vi "passIfError.vi"(6 "passing error codes (default = any error code)":i32[](array[numeric]), 7 "custom report message (\"\")":string, 8 "error in (no error)":errorcluster, 9 "task (\"\")":string, 10 "error":errorcluster, 11 "TestCase in":refnum<class "TestCase.lvclass">) -> (0 "error out":errorcluster, 3 "TestCase out":refnum<class "TestCase.lvclass">)   [LabVIEW 2011, in "TestCase.lvclass"]
doc: "Pass if 'error.status'=TRUE. 'error' is the error generated by the task. 'task' is the description of the task failure. 'error in' is for framework errors not related to the test task. 'passing error codes' can be used to define specific error codes that will cause the test to pass so that unexpected errors are still raised as test failures.\n\nUse this method when you want to test that an expected error is correctly raised."
uses:
  TestCase.lvclass
  TestCase.lvclass/TestCase.ctl
  JKI Reuse/Filter Error Codes (Array)__jki_lib_error_handling -- VI Tester.vi
panel:
  # "JKI VI Tester for LabVIEW\nhttp://jkisoft.com/vi-tester\nCopyright (C) 2007-2009, JKI <info@jkisoft.com>\nALL RIGHTS RESERVED"
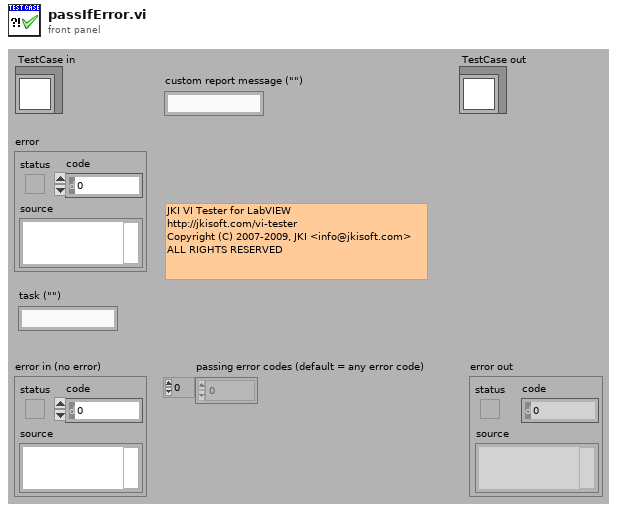
[diagram p1: front panel]
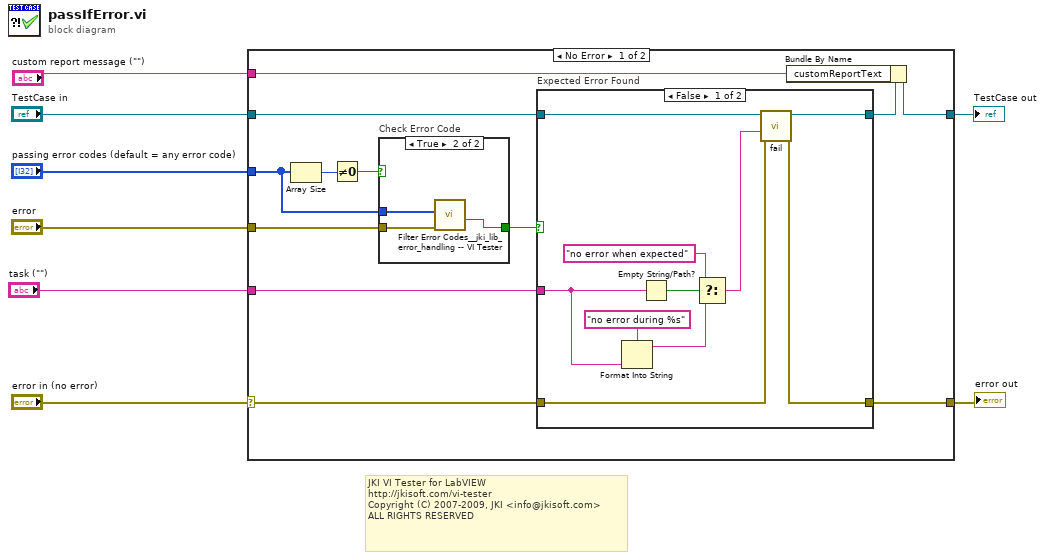
[diagram p0: block diagram]
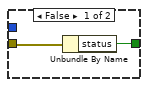
[diagram p2: hidden frame]
diagram:
  # "JKI VI Tester for LabVIEW\nhttp://jkisoft.com/vi-tester\nCopyright (C) 2007-2009, JKI <info@jkisoft.com>\nALL RIGHTS RESERVED"
  n1 = case shown="No Error" "error in (no error)" {
    selector: "error in (no error)" -> [w20 w39]
    tunnel: [w19 w39] -> w7
    tunnel: [w15 w38] -> w5
    tunnel: "TestCase in" -> [w18 w38]
    tunnel: "error" -> [w13 _]
    tunnel: "task (\"\")" -> [w17 _]
    tunnel: "custom report message (\"\")" -> [w14 _]
    tunnel: "passing error codes (default = any error code)" -> [w10 _]
    frame No Error {
      n2 = Array Size(array=w10) -> (size(s)=w9:i32)
      n3 = Not Equal To 0?(x=w9) -> (x != 0?=w12:bool)
      n4 = case "Check Error Code" shown="True" w12 {
        tunnel: w10 -> [_ w25]
        tunnel: w13 -> [w22 w24]
        tunnel: [w21 w23] -> w11
        frame False {
          n5 = Unbundle By Name(w22) -> ("status"=w21:bool)
        }
        frame True {
          n6 = call-poly "Filter Error Codes__jki_lib_error_handling -- VI Tester.vi"("error in"=w24, "error codes to filter"=w25) -> ("error filtered?"=w23:bool)  [unwired: 7 in, 2 out]
        }
      }
      n7 = case "Expected Error Found" shown="False" w11 {
        tunnel: [w34 w37] -> w19
        tunnel: w20 -> [w35 w37]
        tunnel: w18 -> [w33 w36]
        tunnel: [w32 w36] -> w16
        tunnel: w17 -> [w30 _]
        frame False {
          n8 = Format Into String(format string="no error during %s", w30) -> (resulting string=w26:string)  [unwired: 2 in, 1 out]
          n9 = Empty String/Path?(string/path=w30) -> (empty?=w29:bool)
          n10 = Select(t="no error when expected" ("message (\"\")"), s=w29, f=w26) -> (s? t:f=w27:string)
          n11 = call-dynamic "fail.vi"("error in (no error)"=w35, "message (\"\")"=w27, "TestCase in"=w33) -> ("error out"=w34:errorcluster, "TestCase out"=w32:refnum<class "TestCase.lvclass">)  [unwired: 7 in]
        }
        frame True {
          # "do nothing (test passed)"
        }
      }
      n12 = Bundle By Name(cluster=w16, "customReportText"=w14) -> (w15:refnum<class "TestCase.lvclass">)
    }
    frame Error {
    }
  }
  "error out" <- w7
  "TestCase out" <- w5
